vi "App_Main 1.vi"() -> ()   [LabVIEW 2018, in "Application 1.lvlib"]
uses:
  Application 1.lvlib
  Cloud Server/Data Def/Server_Error Handle Method.ctl
  Data Def/App_Subpanel Name.ctl
  Data Def/App_User Event Data.ctl
  Data Def/App_Main Loop Queue Data.ctl
  Data Def/App_Tips Data.ctl
  Cloud Server/Cloud Server.lvlib
panel:
  out "Time":timestamp format="%<%H:%M:%S>T"
  out "Connection?":bool
  out "User Name":string
  out "Login?":bool
  out "Tips":string
  in  "Stop":bool caption="Power"
  in  "Home":bool caption="Menu"
  # "Smart ECG Client"
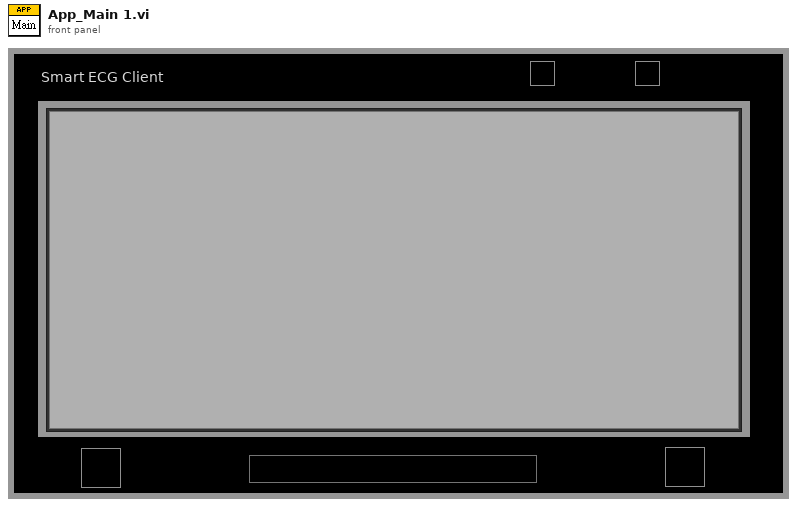
[diagram p1: front panel]
types:
  T1 = typedef "Cloud Server.lvlib/Server_Error Handle Method.ctl" = enum16{"Initialize", "Get Queue Ref.", "Enqueue", "Insert", "Flush", "Release"}
  T2 = typedef "Application 1.lvlib/App_User Event Data.ctl" = cluster{"Command":string, "Data":variant}
  T3 = typedef "Application 1.lvlib/App_Subpanel Name.ctl" = enum16{"Main", "Menu", "User Registering", "User Setting", "Monitor", "Traning Mode", "Query Data", "Connect Setting"}
  T4 = typedef "Application 1.lvlib/App_Main Loop Queue Data.ctl" = cluster{"Command":string, "Data":variant}
  T5 = typedef "Application 1.lvlib/App_Main Data.ctl" = cluster{"VI Refnum":refnum<vi>, "Subpanel":refnum<vi>, "Connection ID":refnum<k5>, "Meta data":T6[], "Main Queue":T8, "User Data":T9}
  T6 = typedef "stm_MetaElement.ctl" = cluster{"Name":T7}
  T7 = typedef "stm_MetaDataElement.ctl" = string
  T8 = typedef "Application 1.lvlib/App_Main Queue.ctl" = cluster{"Main Loop Queue":refnum<queue>}
  T9 = typedef "User Data.ctl" = cluster{"Name":string, "Email":string, "Phone Number":string, "User Picture":u32[][], "Last Login Time":timestamp}
  T10 = typedef "Application 1.lvlib/App_Tips Data.ctl" = cluster{"Tips":string, "BG Color":u32}
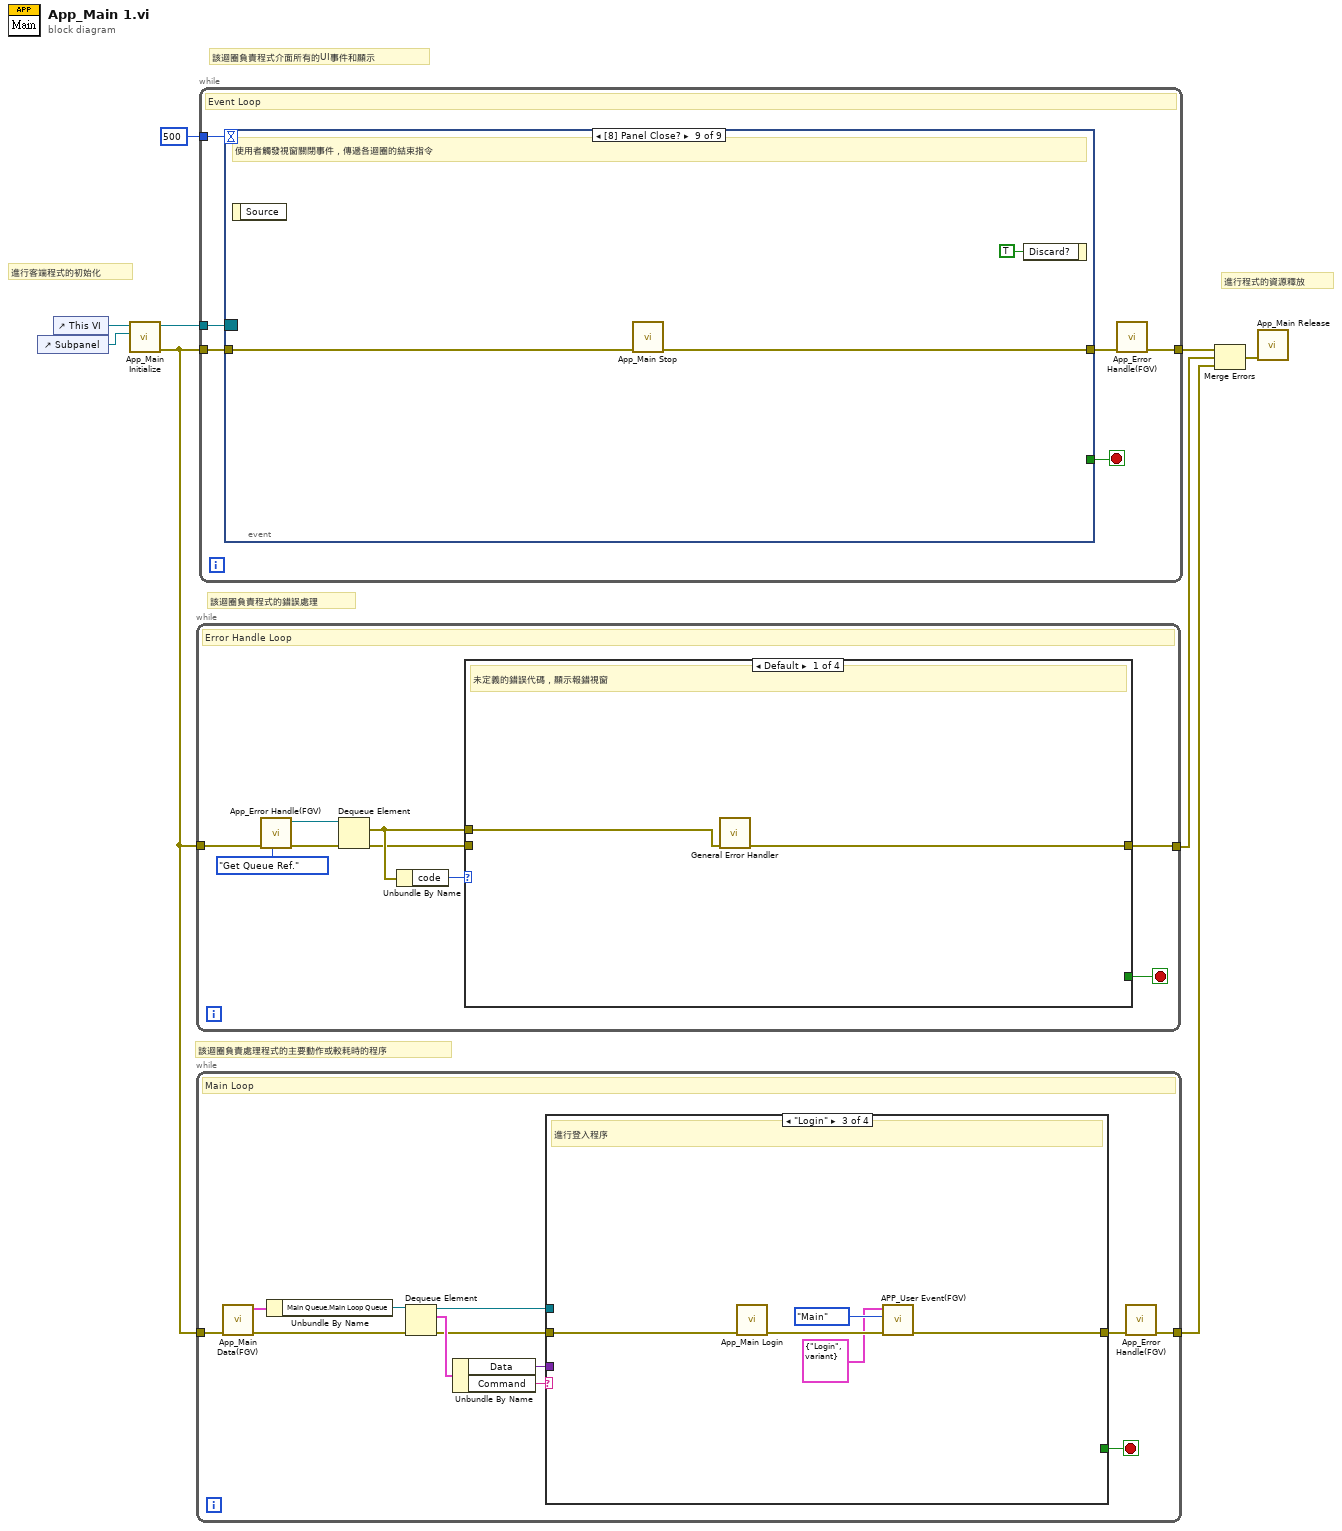
[diagram p0: block diagram]
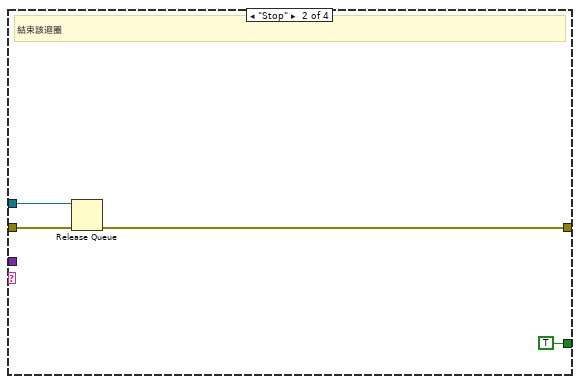
[diagram p3: hidden frame]
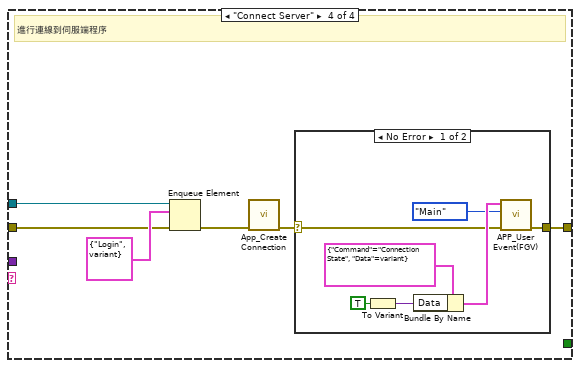
[diagram p4: hidden frame]
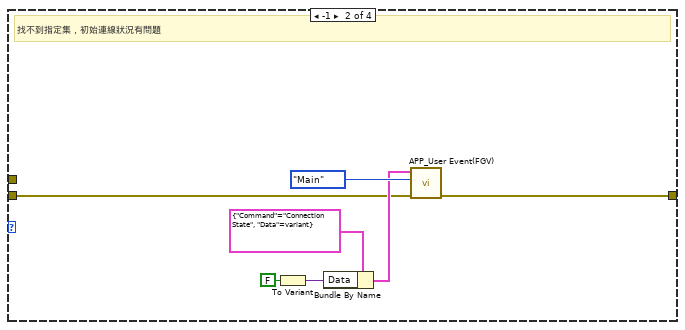
[diagram p6: hidden frame]
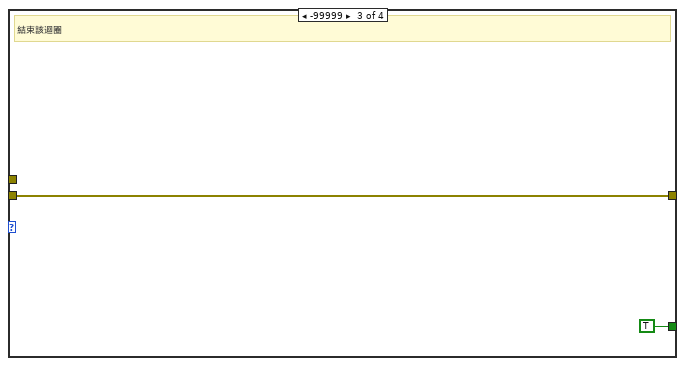
[diagram p7: hidden frame]
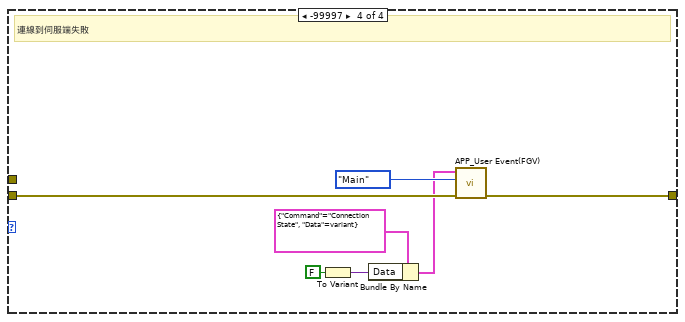
[diagram p8: hidden frame]
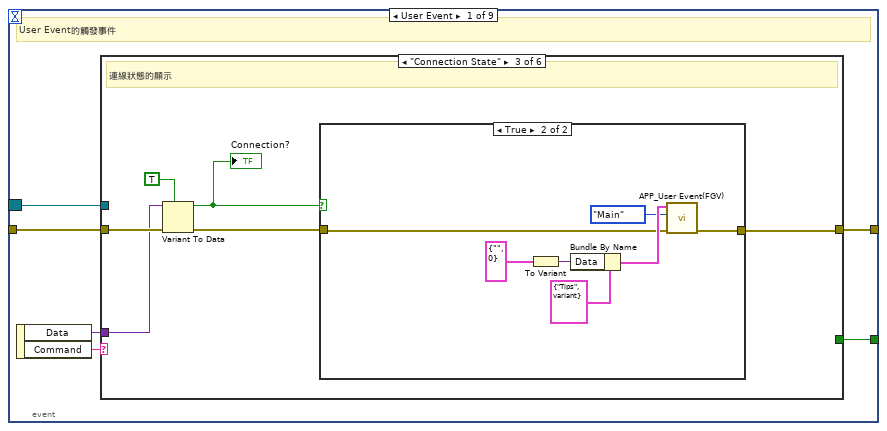
[diagram p9: hidden frame]
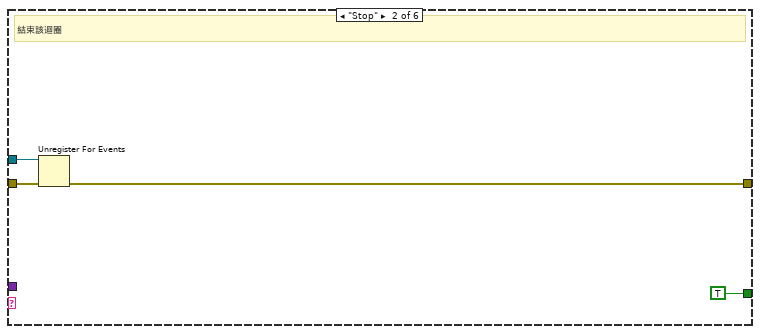
[diagram p11: hidden frame]
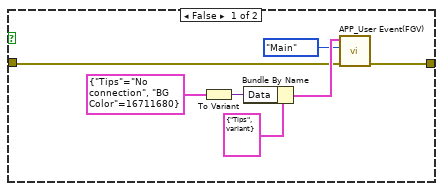
[diagram p12: hidden frame]
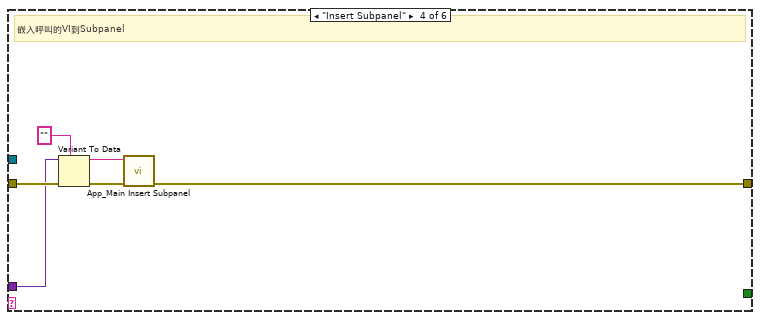
[diagram p13: hidden frame]
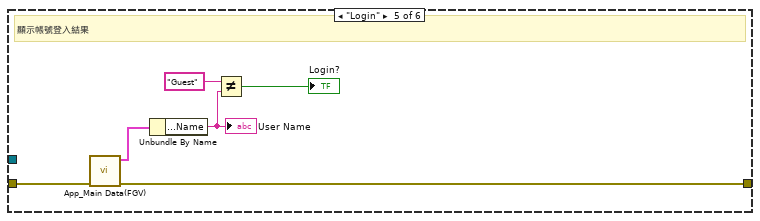
[diagram p14: hidden frame]
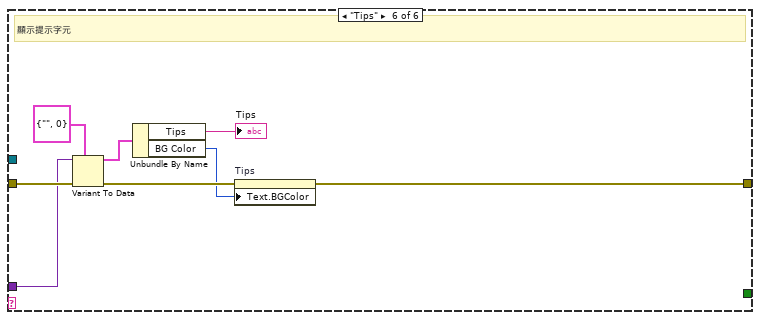
[diagram p15: hidden frame]
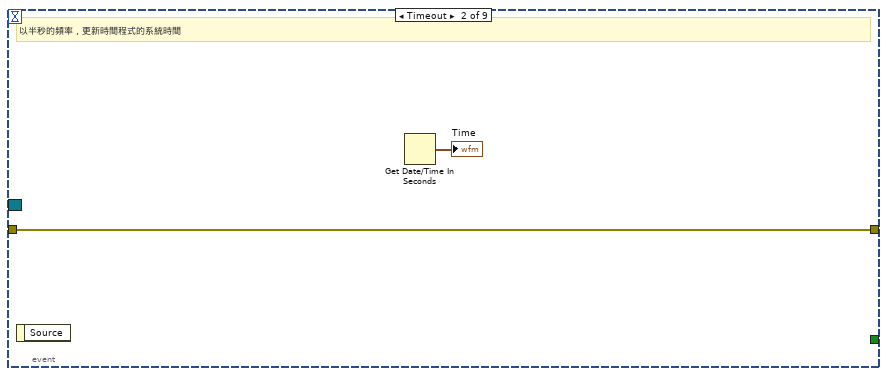
[diagram p16: hidden frame]
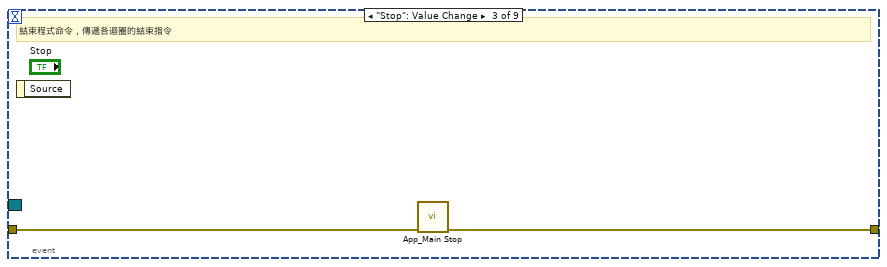
[diagram p17: hidden frame]
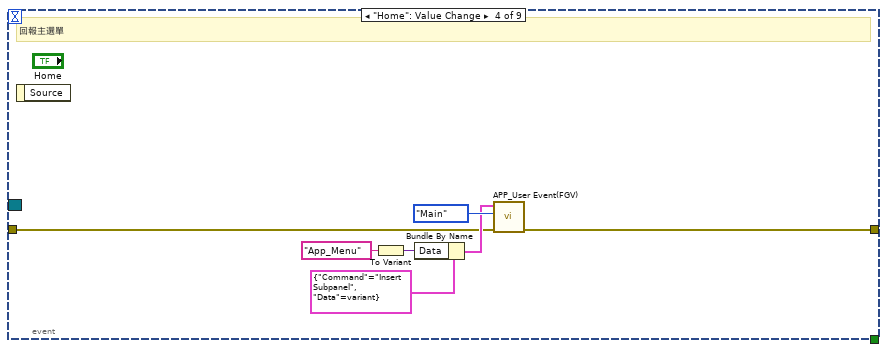
[diagram p18: hidden frame]
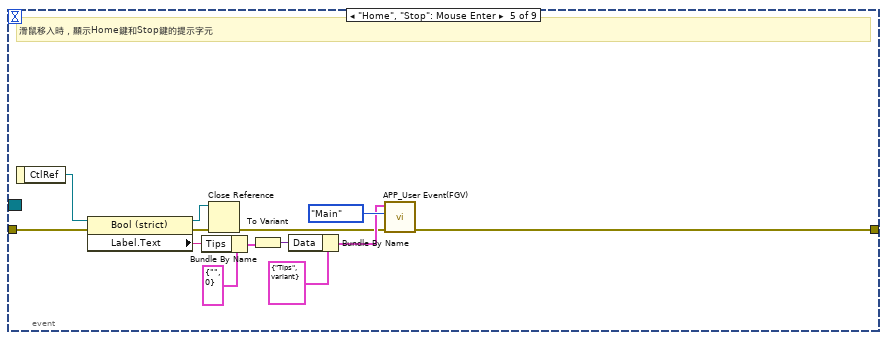
[diagram p19: hidden frame]
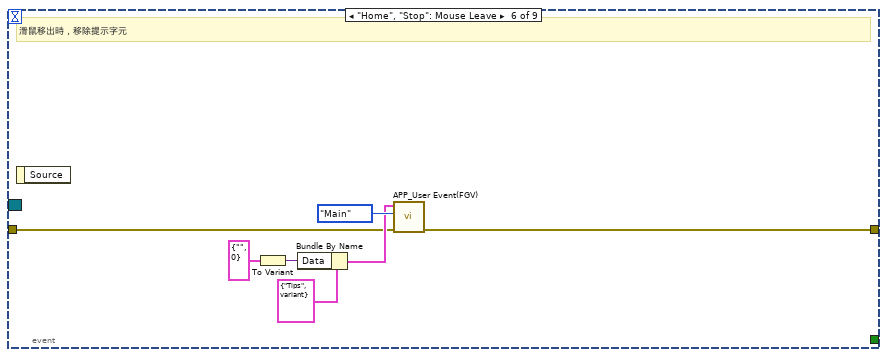
[diagram p20: hidden frame]
diagram:
  # "進行程式的資源釋放"
  # "該迴圈負責處理程式的主要動作或較耗時的程序"
  # "該迴圈負責程式的錯誤處理"
  # "該迴圈負責程式介面所有的UI事件和顯示"
  # "進行客端程式的初始化"
  n1 = control-ref of="Subpanel"() -> (w7:refnum<vi>)
  n2 = control-ref of="This VI"() -> (w9:refnum<vi>)
  n3 = call "App_Main Initialize.vi"("Subpanel"=w7, "VI Reference"=w9) -> ("error out"=w2:errorcluster, "Event Registration Refnum"=w8:refnum<event-registration>)  [unwired: 8 in]
  n4 = while {
    tunnel: w2 -> [w18]
    tunnel: [w10] -> w4
    stop <- w11 stop-if-true
    # "Error Handle Loop"
    n5 = call "App_Error Handle(FGV).vi"("Error Handle Method(Enqueue)"=Server_Error_Handle_Method."Get Queue Ref.", "error in"=w18) -> ("error out"=w16:errorcluster, "Queue Ref."=w15:refnum<queue>)  [unwired: 8 in]
    n6 = Dequeue Element(queue=w15, error in (no error)=w16) -> (element=w13:errorcluster, error out=w12:errorcluster)  [unwired: 1 in, 2 out]
    n7 = Unbundle By Name(w13) -> ("code"=w14:i32)
    n8 = case shown="Default" w14 {
      tunnel: w13 -> [w20 _ _ _]
      tunnel: w12 -> [_ w22 w28 w35]
      tunnel: [_ _ TRUE _] -> w11
      tunnel: [w19 w21 w28 w30] -> w10
      frame Default {
        # "未定義的錯誤代碼，顯示報錯視窗"
        n9 = call <vilib>:"General Error Handler.vi"("error in (no error)"=w20) -> ("error out"=w19:errorcluster)  [unwired: 10 in, 4 out]
      }
      frame -1 {
        # "找不到指定集，初始連線狀況有問題"
        n10 = To Variant(anything=FALSE) -> (Variant=w25:variant)
        n11 = Bundle By Name(cluster=T2 {"Command"="Connection State", "Data"=variant} ("User Event Data"), "Data"=w25) -> (w23:T2)
        n12 = call "APP_User Event(FGV).vi"("error in"=w22, "Subpanel Name"=App_Subpanel_Name."Main", "User Event Data"=w23) -> ("error out"=w21:errorcluster)  [unwired: 7 in, 1 out]
      }
      frame -99999 {
        # "結束該迴圈"
      }
      frame -99997 {
        # "連線到伺服端失敗"
        n13 = To Variant(anything=FALSE) -> (Variant=w33:variant)
        n14 = Bundle By Name(cluster=T2 {"Command"="Connection State", "Data"=variant} ("User Event Data"), "Data"=w33) -> (w31:T2)
        n15 = call "APP_User Event(FGV).vi"("error in"=w35, "Subpanel Name"=App_Subpanel_Name."Main", "User Event Data"=w31) -> ("error out"=w30:errorcluster)  [unwired: 7 in, 1 out]
      }
    }
  }
  n16 = while {
    tunnel: w2 -> [w48]
    tunnel: [w39] -> w1
    stop <- w37 stop-if-true
    # "Main Loop"
    n17 = call "App_Main Data(FGV).vi"("error in"=w48) -> ("error out"=w46:errorcluster, "Main Data Out"=w47:T5)  [unwired: 9 in]
    n18 = Unbundle By Name(w47) -> ("Main Queue.Main Loop Queue"=w45:refnum<queue>)
    n19 = Dequeue Element(queue=w45, error in (no error)=w46) -> (queue out=w38:refnum<queue>, element=w44:T4, error out=w41:errorcluster)  [unwired: 1 in, 1 out]
    n20 = Unbundle By Name(w44) -> ("Data"=w42:variant, "Command"=w43:string)
    n21 = case shown="\"Login\"" w43 {
      tunnel: w42 -> [_ _ _ _]
      tunnel: w41 -> [w49 w53 w58 w61]
      tunnel: [w49 w51 w54 w63] -> w40
      tunnel: w38 -> [_ w52 _ w59]
      tunnel: [_ TRUE _ _] -> w37
      frame Default {
        # "未定義的命令"
      }
      frame "Stop" {
        # "結束該迴圈"
        n22 = Release Queue(queue=w52, error in (no error)=w53) -> (error out=w51:errorcluster)  [unwired: 1 in, 2 out]
      }
      frame "Login" {
        # "進行登入程序"
        n23 = call "App_Main Login.vi"("error in"=w58) -> ("error out"=w56:errorcluster)  [unwired: 10 in]
        n24 = call "APP_User Event(FGV).vi"("error in"=w56, "Subpanel Name"=App_Subpanel_Name."Main", "User Event Data"=T2 {"Command"="Login", "Data"=variant}) -> ("error out"=w54:errorcluster)  [unwired: 7 in, 1 out]
      }
      frame "Connect Server" {
        # "進行連線到伺服端程序"
        n25 = Enqueue Element(queue=w59, element=T4 {"Command"="Login", "Data"=variant}, error in (no error)=w61) -> (error out=w60:errorcluster)  [unwired: 1 in, 2 out]
        n26 = call "App_Create Connection.vi"("error in"=w60) -> ("error out"=w64:errorcluster)  [unwired: 10 in]
        n27 = case shown="No Error" w64 {
          selector: w64 -> [w66 w72]
          tunnel: [w65 w72] -> w63
          frame No Error {
            n28 = To Variant(anything=TRUE) -> (Variant=w69:variant)
            n29 = Bundle By Name(cluster=T2 {"Command"="Connection State", "Data"=variant} ("User Event Data"), "Data"=w69) -> (w71:T2)
            n30 = call "APP_User Event(FGV).vi"("error in"=w66, "Subpanel Name"=App_Subpanel_Name."Main", "User Event Data"=w71) -> ("error out"=w65:errorcluster)  [unwired: 7 in, 1 out]
          }
          frame Error {
          }
        }
      }
    }
    n31 = call "App_Error Handle(FGV).vi"("error in"=w40) -> ("error out"=w39:errorcluster)  [unwired: 9 in, 1 out]
  }
  n32 = while {
    tunnel: w2 -> [w77]
    tunnel: w8 -> [w78]
    tunnel: [w74] -> w5
    tunnel: 500 -> [w73]
    stop <- w76 stop-if-true
    # "Event Loop"
    n33 = event shown="[8] Panel Close?" {
      selector: w78 -> [w81 _ _ _ _ _ _ _ _]
      dyn-events: _ -> [_ _ _ _ _ _ _ _ _]
      timeout: w73 -> [_ _ _ _ _ _ _ _ _]
      tunnel: w77 -> [w82 w130 w133 w135 w153 w156 w164 w169 w183]
      tunnel: [w80 w130 w132 w134 w144 w155 w163 w168 w182] -> w75
      tunnel: [w79 _ _ _ _ _ _ _ _] -> w76
      event User Event {
        # "User Event的觸發事件"
        n34 = event-data() -> ("Data"=w83:variant, "Command"=w84:string)  [unwired: 1 in]
        n35 = case shown="\"Connection State\"" w84 {
          tunnel: w83 -> [_ _ w94 w114 _ w128]
          tunnel: w82 -> [w85 w89 w95 w115 w121 w129]
          tunnel: w81 -> [_ w88 _ _ _ _]
          tunnel: [w85 w87 w90 w110 w119 w126] -> w80
          tunnel: [_ TRUE _ _ _ _] -> w79
          frame Default {
            # "未定義的命令"
          }
          frame "Stop" {
            # "結束該迴圈"
            n36 = Unregister For Events(event registration refnum=w88, error in=w89) -> (error out=w87:errorcluster)
          }
          frame "Connection State" {
            # "連線狀態的顯示"
            n37 = Variant To Data(error in=w95, type=TRUE, Variant=w94) -> (data=w91:bool, error out=w92:errorcluster)
            "Connection?" <- w91
            n38 = case shown="True" w91 {
              tunnel: w92 -> [w97 w104]
              tunnel: [w96 w103] -> w90
              frame False {
                n39 = To Variant(anything=T10 {"Tips"="No connection", "BG Color"=16711680} ("Tips Data")) -> (Variant=w100:variant)
                n40 = Bundle By Name(cluster=T2 {"Command"="Tips", "Data"=variant} ("User Event Data"), "Data"=w100) -> (w101:T2)
                n41 = call "APP_User Event(FGV).vi"("error in"=w97, "Subpanel Name"=App_Subpanel_Name."Main", "User Event Data"=w101) -> ("error out"=w96:errorcluster)  [unwired: 7 in, 1 out]
              }
              frame True {
                n42 = To Variant(anything=T10 {"Tips"="", "BG Color"=0} ("Tips Data")) -> (Variant=w107:variant)
                n43 = Bundle By Name(cluster=T2 {"Command"="Tips", "Data"=variant} ("User Event Data"), "Data"=w107) -> (w108:T2)
                n44 = call "APP_User Event(FGV).vi"("error in"=w104, "Subpanel Name"=App_Subpanel_Name."Main", "User Event Data"=w108) -> ("error out"=w103:errorcluster)  [unwired: 7 in, 1 out]
              }
            }
          }
          frame "Insert Subpanel" {
            # "嵌入呼叫的VI到Subpanel"
            n45 = Variant To Data(error in=w115, type="", Variant=w114) -> (data=w111:string, error out=w112:errorcluster)
            n46 = call "App_Main Insert Subpanel.vi"("error in"=w112, "VI Name"=w111) -> ("error out"=w110:errorcluster)  [unwired: 9 in]
          }
          frame "Login" {
            # "顯示帳號登入結果"
            n47 = call "App_Main Data(FGV).vi"("error in"=w121) -> ("error out"=w119:errorcluster, "Main Data Out"=w120:T5)  [unwired: 9 in]
            n48 = Unbundle By Name(w120) -> ("User Data.Name"=w118:string)
            "User Name" <- w118
            n49 = Not Equal?(x="Guest", y=w118) -> (x != y?=→"Login?":bool)
          }
          frame "Tips" {
            # "顯示提示字元"
            n50 = Variant To Data(error in=w129, type=T10 {"Tips"="", "BG Color"=0} ("Tips Data"), Variant=w128) -> (data=w124:T10, error out=w127:errorcluster)
            n51 = Unbundle By Name(w124) -> ("Tips"=→"Tips":string, "BG Color"=w122:u32)
            n52 = property on="Tips" class="Str"(error in=w127, "Text.BGColor"=w122) -> (error out=w126:errorcluster)  [unwired: 1 in, 1 out]
          }
        }
      }
      event Timeout {
        # "以半秒的頻率，更新時間程式的系統時間"
        n53 = event-data() -> ()  [unwired: 1 in, 1 out]
        n54 = Get Date/Time In Seconds() -> (seconds since 1Jan1904=→"Time":timestamp)
      }
      event "Stop": Value Change {
        # "結束程式命令，傳遞各迴圈的結束指令"
        n55 = event-data() -> ()  [unwired: 1 in, 1 out]
        n56 = call "App_Main Stop.vi"("error in"=w133) -> ("error out"=w132:errorcluster)  [unwired: 10 in]
      }
      event "Home": Value Change {
        # "回報主選單"
        n57 = event-data() -> ()  [unwired: 1 in, 1 out]
        n58 = To Variant(anything="App_Menu") -> (Variant=w138:variant)
        n59 = Bundle By Name(cluster=T2 {"Command"="Insert Subpanel", "Data"=variant} ("User Event Data"), "Data"=w138) -> (w136:T2)
        n60 = call "APP_User Event(FGV).vi"("error in"=w135, "Subpanel Name"=App_Subpanel_Name."Main", "User Event Data"=w136) -> ("error out"=w134:errorcluster)  [unwired: 7 in, 1 out]
      }
      event "Home", "Stop": Mouse Enter {
        # "滑鼠移入時，顯示Home鍵和Stop鍵的提示字元"
        n61 = event-data() -> ("CtlRef"=w152:refnum<vi>)  [unwired: 1 in]
        n62 = property class="Bool (strict)"(reference=w152, error in=w153) -> (reference out=w146:refnum<vi>, error out=w147:errorcluster, "Label.Text"=w142:string)
        n63 = Bundle By Name(cluster=T10 {"Tips"="", "BG Color"=0} ("Tips Data"), "Tips"=w142) -> (w143:T10)
        n64 = Close Reference(reference=w146, error in (no error)=w147) -> (error out=w145:errorcluster)
        n65 = To Variant(anything=w143) -> (Variant=w149:variant)
        n66 = Bundle By Name(cluster=T2 {"Command"="Tips", "Data"=variant} ("User Event Data"), "Data"=w149) -> (w148:T2)
        n67 = call "APP_User Event(FGV).vi"("error in"=w145, "Subpanel Name"=App_Subpanel_Name."Main", "User Event Data"=w148) -> ("error out"=w144:errorcluster)  [unwired: 7 in, 1 out]
      }
      event "Home", "Stop": Mouse Leave {
        # "滑鼠移出時，移除提示字元"
        n68 = event-data() -> ()  [unwired: 1 in, 1 out]
        n69 = To Variant(anything=T10 {"Tips"="", "BG Color"=0} ("Tips Data")) -> (Variant=w158:variant)
        n70 = Bundle By Name(cluster=T2 {"Command"="Tips", "Data"=variant} ("User Event Data"), "Data"=w158) -> (w157:T2)
        n71 = call "APP_User Event(FGV).vi"("error in"=w156, "Subpanel Name"=App_Subpanel_Name."Main", "User Event Data"=w157) -> ("error out"=w155:errorcluster)  [unwired: 7 in, 1 out]
      }
      event "Connection?": Mouse Up {
        # "點選連線狀態時，將Subpanel嵌入負責連線設定功能的VI"
        n72 = event-data() -> ()  [unwired: 1 in, 1 out]
        n73 = To Variant(anything="App_Connect Setting") -> (Variant=w162:variant)
        n74 = Bundle By Name(cluster=T2 {"Command"="Insert Subpanel", "Data"=variant} ("User Event Data"), "Data"=w162) -> (w165:T2)
        n75 = call "APP_User Event(FGV).vi"("error in"=w164, "Subpanel Name"=App_Subpanel_Name."Main", "User Event Data"=w165) -> ("error out"=w163:errorcluster)  [unwired: 7 in, 1 out]
      }
      event "Login?": Mouse Up {
        # "點選登入狀態時，如果已登入則顯示帳號資訊，如果未登入則顯示帳號註冊"
        n76 = event-data() -> ()  [unwired: 1 in, 1 out]
        n77 = call "App_Main Data(FGV).vi"("error in"=w169) -> ("error out"=w176:errorcluster, "Main Data Out"=w175:T5)  [unwired: 9 in]
        n78 = Unbundle By Name(w175) -> ("User Data.Name"=w173:string)
        n79 = Not Equal?(x="Guest", y=w173) -> (x != y?=w172:bool)
        n80 = Select(t="App_User Setting", s=w172, f="App_User Registering") -> (s? t:f=w177:string)
        n81 = To Variant(anything=w177) -> (Variant=w180:variant)
        n82 = Bundle By Name(cluster=T2 {"Command"="Insert Subpanel", "Data"=variant} ("User Event Data"), "Data"=w180) -> (w178:T2)
        n83 = call "APP_User Event(FGV).vi"("error in"=w176, "Subpanel Name"=App_Subpanel_Name."Main", "User Event Data"=w178) -> ("error out"=w168:errorcluster)  [unwired: 7 in, 1 out]
      }
      event Panel Close? {
        # "使用者觸發視窗關閉事件，傳遞各迴圈的結束指令"
        n84 = event-data() -> ()  [unwired: 1 in, 1 out]
        n85 = call "App_Main Stop.vi"("error in"=w183) -> ("error out"=w182:errorcluster)  [unwired: 10 in]
        n86 = event-data("Discard?"=TRUE) -> ()  [unwired: 1 in, 1 out]
      }
    }
    n87 = call "App_Error Handle(FGV).vi"("error in"=w75) -> ("error out"=w74:errorcluster)  [unwired: 9 in, 1 out]
  }
  n88 = Merge Errors(w5, w4, w1) -> (w3:errorcluster)
  n89 = call "App_Main Release.vi"("error in"=w3) -> ()  [unwired: 10 in, 1 out]
